vi "daqio_Get_All_Files.vi"(8 "error in (no error)":errorcluster, 11 "daq.io type in":T2={"daq.io ref"=refnum, "daq.io API Base"="http://dashboard.daq.io/api/v1", "Device Key"="", "Account ID"="", "online"=TRUE, "SSL"=TRUE, "buffer"=TRUE}) -> (0 "error out":errorcluster, 2 "Existing Files":T1[](array[typedef]), 3 "daq.io type out":T2={"daq.io ref"=refnum, "daq.io API Base"="http://dashboard.daq.io/api/v1", "Device Key"="", "Account ID"="", "online"=TRUE, "SSL"=TRUE, "buffer"=TRUE})   [LabVIEW 2013, in "daqio minimal.lvlib"]
doc: "This VI retrieves all existing files for the logged in user. To store these files locally, use the \"Save File\" VI."
uses:
  daqio minimal.lvlib
  _typedefs/daqio-Type.ctl
  <vilib>/httpClient/ClientHandle.ctl
  _typedefs/daqio-File.ctl
  <vilib>/Easy HTTP Client/Easy HTTP.lvlib
  <vilib>/httpClient/LabVIEWHTTPClient.lvlib
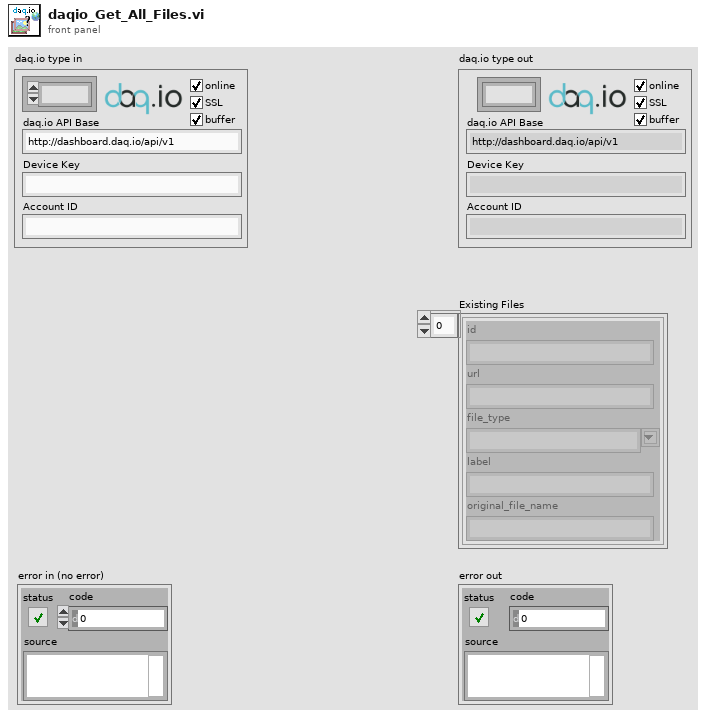
[diagram p1: front panel]
types:
  T1 = typedef "daqio minimal.lvlib/daqio-File.ctl" = cluster{"id":string, "url":string, "file_type":string, "label":string, "original_file_name":string}
  T2 = typedef "daqio minimal.lvlib/daqio-Type.ctl" = cluster{"daq.io ref":T3, "daq.io API Base":string, "Device Key":string, "Account ID":string, "online":bool, "SSL":bool, "buffer":bool}
  T3 = typedef "LabVIEWHTTPClient.lvlib/ClientHandle.ctl" = refnum<k1>
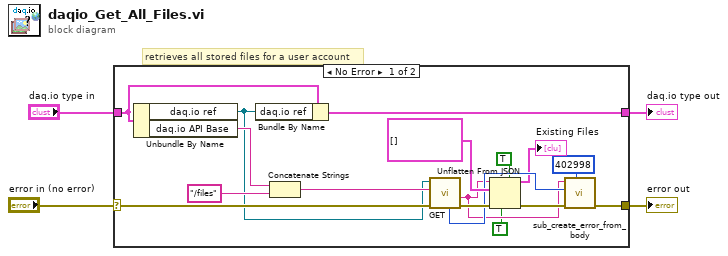
[diagram p0: block diagram]
diagram:
  # "retrieves all stored files for a user account"
  n1 = case shown="No Error" "error in (no error)" {
    selector: "error in (no error)" -> [w16 w22]
    tunnel: "daq.io type in" -> [w18 w23]
    tunnel: [w17 w23] -> w3
    tunnel: [w20 w22] -> w2
    frame No Error {
      n2 = Unbundle By Name(w18) -> ("daq.io ref"=w9:T3, "daq.io API Base"=w19:string)
      n3 = Bundle By Name(cluster=w18, "daq.io ref"=w9) -> (w17:T2)
      n4 = Concatenate Strings(w19, "/files") -> (w14:string)
      n5 = call <vilib>:"GET.vi"("error in (no error)"=w16, "url"=w14, "client handle"=w9) -> ("error out"=w15:errorcluster, "body"=w8:string, "HTTP Response Code"=w11:i32)  [unwired: 4 in, 2 out]
      n6 = Unflatten From JSON(enable LabVIEW extensions? (T)=TRUE, JSON string=w8, type and defaults=T1[] [], default null elements? (F)=TRUE, error in (no error)=w15) -> (value=→"Existing Files":T1[], error out=w12:errorcluster)  [unwired: 2 in]
      n7 = call "sub_create_error_from_body.vi"("error code"=402998, "error in (no error)"=w12, "http code"=w11, "body"=w8) -> ("error out"=w20:errorcluster)  [unwired: 7 in]
    }
    frame Error {
    }
  }
  "error out" <- w2
  "daq.io type out" <- w3
